vi "IGM402_Read.vi"() -> ()   [LabVIEW 2011]
uses:
  <vilib>/Instr/_visa.llb/VISA Configure Serial Port (Instr).vi
panel:
  in  "He3 Correction on IG?":bool
  out "Pressure Chart":dynamicdata(graph)
  in  "Write to File?":bool=TRUE
  out "Time":string
  out "IG buffer":string
  out "CG2 buffer":string
  out "CG1 buffer":string
  out "CG2":dbl
  out "CG1":dbl
  out "IG":dbl
  in  "CG2?":bool
  in  "CG1?":bool
  in  "IG?":bool
  in  "CG2 write string":string="#01RDCG2\r"
  in  "CG1 write string":string="#01RDCG1\r"
  in  "milliseconds wait":u32=3000
  in  "stop":bool
  in  "IG write string":string="#01RD\r"
  in  "VISA resource name":refnum<visa-resource-name>="COM3"
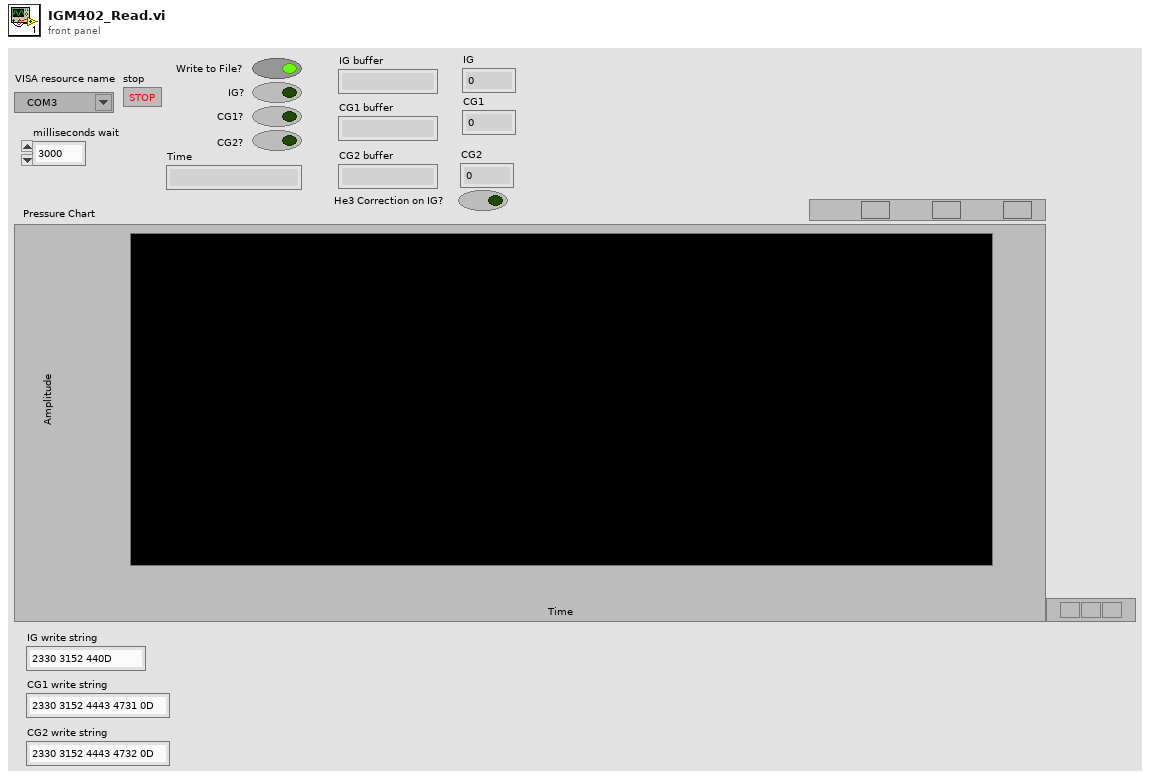
[diagram p1: front panel]
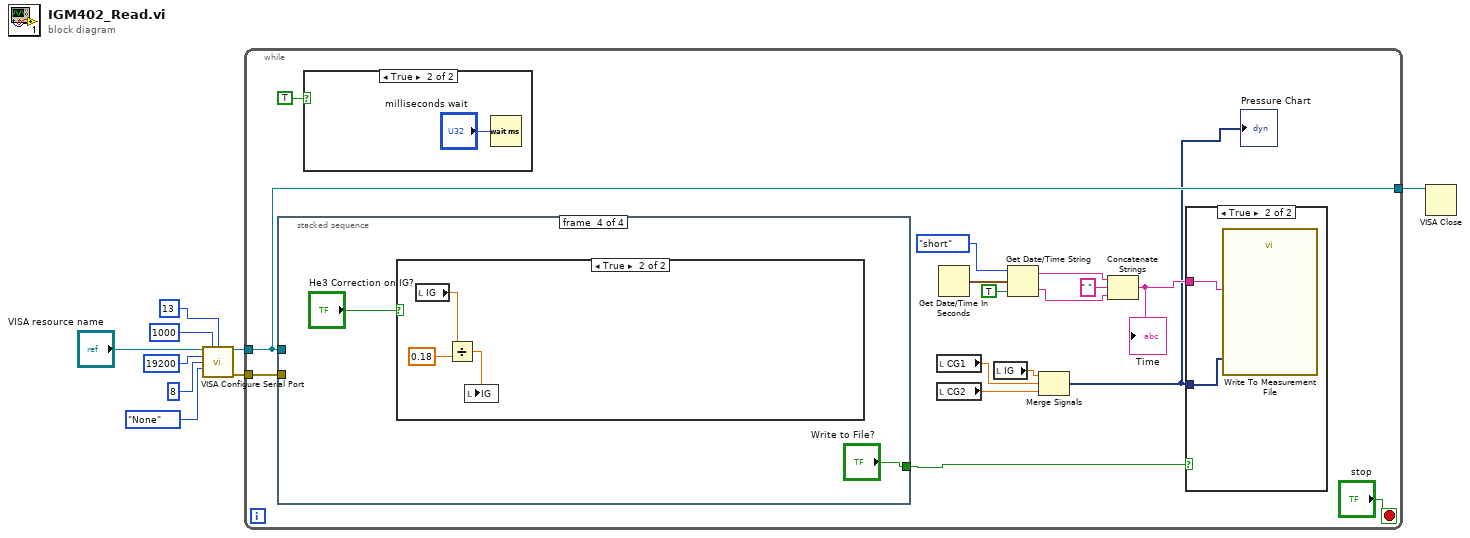
[diagram p0: block diagram]
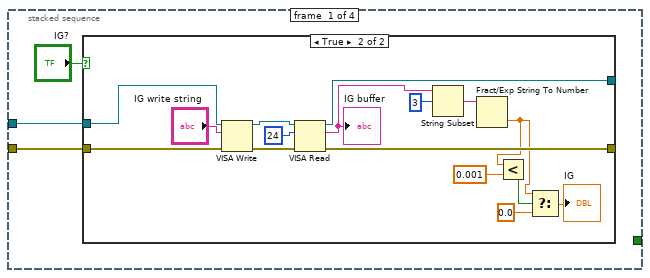
[diagram p3: hidden frame]
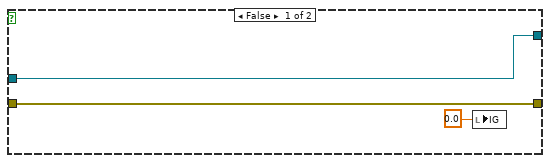
[diagram p4: hidden frame]
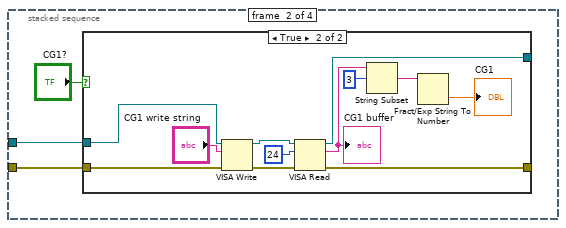
[diagram p5: hidden frame]
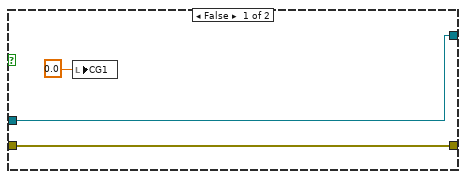
[diagram p6: hidden frame]
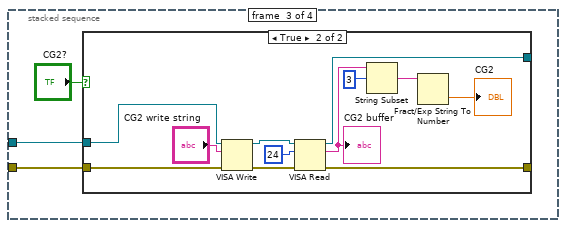
[diagram p7: hidden frame]
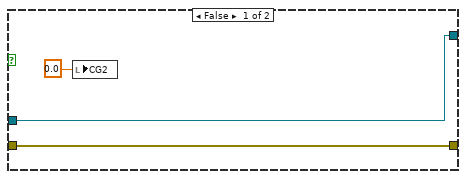
[diagram p8: hidden frame]
diagram:
  n1 = call-poly "VISA Configure Serial Port"("VISA resource name"="VISA resource name", "timeout (10sec)"=u32 1000, "termination char\n(0xA = '\\n' = LF)"=u8 13 ("termination char\n(0xA = '\\n' = LF)"), "baud rate (9600)"=u32 19200, "data bits (8)"=u16 8, "parity (0:none)"=enum16{"None", "Odd", "Even", "Mark", "Space"}."None") -> ("VISA resource name out"=w9:refnum<visa-resource-name>, "error out"=w8:errorcluster)  [unwired: 8 in]
  n2 = while {
    tunnel: w9 -> [w22]
    tunnel: w8 -> [w23]
    tunnel: [w22] -> w1
    stop <- "stop" stop-if-true
    n3 = stacked-sequence {
      tunnel: w22 -> [w30 w52 w70 _]
      tunnel: w23 -> [w28 w50 w68 _]
      tunnel: [_ _ _ "Write to File?"] -> w10
      frame #0 {
        n4 = case shown="True" "IG?" {
          tunnel: w30 -> [w33 w49]
          tunnel: [w33 w42] -> _
          tunnel: w28 -> [w32 w48]
          tunnel: [w32 w40] -> _
          frame False {
            n5 = local write "IG"(0.0 ("IG")) -> ()
          }
          frame True {
            n6 = VISA Write(VISA resource name=w49, write buffer="IG write string", error in (no error)=w48) -> (VISA resource name out=w43:refnum<visa-resource-name>, error out=w41:errorcluster)  [unwired: 1 out]
            n7 = VISA Read(VISA resource name=w43, byte count=u32 24, error in (no error)=w41) -> (VISA resource name out=w42:refnum<visa-resource-name>, read buffer=w44:string, error out=w40:errorcluster)  [unwired: 1 out]
            "IG buffer" <- w44
            n8 = String Subset(string=w44, offset (0)=3) -> (substring=w45:string)  [unwired: 1 in]
            n9 = Fract/Exp String To Number(string=w45) -> (number=w35:dbl)  [unwired: 3 in, 1 out]
            n10 = Less?(x=w35, y=0.001) -> (x < y?=w36:bool)
            n11 = Select(t=w35, s=w36, f=0.0) -> (s? t:f=→"IG":dbl)
          }
        }
      }
      frame #1 {
        n12 = case shown="True" "CG1?" {
          tunnel: w52 -> [w55 w67]
          tunnel: [w55 w60] -> _
          tunnel: w50 -> [w54 w66]
          tunnel: [w54 w58] -> _
          frame False {
            n13 = local write "CG1"(0.0 ("CG1 2")) -> ()
          }
          frame True {
            n14 = VISA Write(VISA resource name=w67, write buffer="CG1 write string", error in (no error)=w66) -> (VISA resource name out=w61:refnum<visa-resource-name>, error out=w59:errorcluster)  [unwired: 1 out]
            n15 = VISA Read(VISA resource name=w61, byte count=u32 24, error in (no error)=w59) -> (VISA resource name out=w60:refnum<visa-resource-name>, read buffer=w62:string, error out=w58:errorcluster)  [unwired: 1 out]
            "CG1 buffer" <- w62
            n16 = String Subset(string=w62, offset (0)=3) -> (substring=w63:string)  [unwired: 1 in]
            n17 = Fract/Exp String To Number(string=w63) -> (number=→"CG1":dbl)  [unwired: 3 in, 1 out]
          }
        }
      }
      frame #2 {
        n18 = case shown="True" "CG2?" {
          tunnel: w70 -> [w73 w85]
          tunnel: [w73 w79] -> _
          tunnel: w68 -> [w72 w84]
          tunnel: [w72 w78] -> _
          frame False {
            n19 = local write "CG2"(0.0 ("CG2")) -> ()
          }
          frame True {
            n20 = VISA Write(VISA resource name=w85, write buffer="CG2 write string", error in (no error)=w84) -> (VISA resource name out=w81:refnum<visa-resource-name>, error out=w80:errorcluster)  [unwired: 1 out]
            n21 = VISA Read(VISA resource name=w81, byte count=u32 24, error in (no error)=w80) -> (VISA resource name out=w79:refnum<visa-resource-name>, read buffer=w75:string, error out=w78:errorcluster)  [unwired: 1 out]
            "CG2 buffer" <- w75
            n22 = String Subset(string=w75, offset (0)=3) -> (substring=w76:string)  [unwired: 1 in]
            n23 = Fract/Exp String To Number(string=w76) -> (number=→"CG2":dbl)  [unwired: 3 in, 1 out]
          }
        }
      }
      frame #3 {
        n24 = case shown="True" "He3 Correction on IG?" {
          frame False {
          }
          frame True {
            n25 = local read "IG"() -> (w89:dbl)
            n26 = Divide(x=w89, y=0.18) -> (x/y=w90:dbl)
            n27 = local write "IG"(w90) -> ()
          }
        }
      }
    }
    n28 = case shown="True" TRUE {
      frame False {
      }
      frame True {
        n29 = Wait (ms)(milliseconds to wait="milliseconds wait") -> ()  [unwired: 1 out]
      }
    }
    n30 = local read "CG1"() -> (w14:dbl)
    n31 = local read "CG2"() -> (w13:dbl)
    n32 = Get Date/Time In Seconds() -> (seconds since 1Jan1904=w16:timestamp)
    n33 = local read "IG"() -> (w15:dbl)
    n34 = Get Date/Time String(date format (0)=enum16{"short", "long", "abbreviated"}."short", seconds (now)=w16, want seconds? (F)=TRUE) -> (date string=w19:string, time string=w18:string)
    n35 = Merge Signals(w15, w14, w13) -> (w11:dynamicdata)
    "Pressure Chart" <- w11
    n36 = Concatenate Strings(w19, " " ("string"), w18) -> (w12:string)
    "Time" <- w12
    n37 = case shown="True" w10 {
      tunnel: w12 -> [_ w27]
      tunnel: w11 -> [_ w26]
      frame False {
      }
      frame True {
        n38 = call "Write To Measurement File"("Signals"=w26, "Comment"=w27) -> ()  [unwired: 15 in, 3 out]
      }
    }
  }
  n39 = VISA Close(VISA resource name=w1) -> ()  [unwired: 1 in, 1 out]
